vi "Write to Pivots.vi"   [LabVIEW 2014]
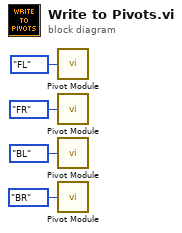
[diagram p0: block diagram]
diagram:
  n1 = call "Pivot Module.vi"("pivot"=enum16{"FL", "FR", "BL", "BR"}."FL") -> ()
  n2 = call "Pivot Module.vi"("pivot"=enum16{"FL", "FR", "BL", "BR"}."FR") -> ()
  n3 = call "Pivot Module.vi"("pivot"=enum16{"FL", "FR", "BL", "BR"}."BL") -> ()
  n4 = call "Pivot Module.vi"("pivot"=enum16{"FL", "FR", "BL", "BR"}."BR") -> ()
